vi "GetElevatorStatus.vi"(11 "Action":enum16{"Get", "Set", "Clear"}(ring)) -> (3 "Elevator Done?":bool)   [LabVIEW 2014, in "Elevator System.lvlib"]
uses:
  Elevator System.lvlib
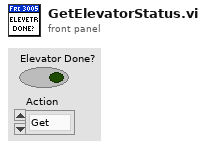
[diagram p1: front panel]
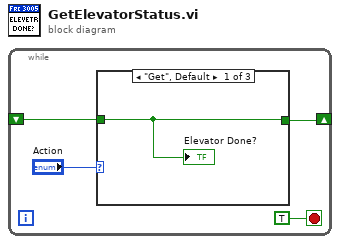
[diagram p0: block diagram]
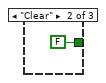
[diagram p2: hidden frame]
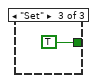
[diagram p3: hidden frame]
diagram:
  n1 = while {
    shift-right: [w2] -> _
    shift-left: _ -> [w1]
    stop <- TRUE stop-if-true
    n2 = case shown="\"Get\", Default" "Action" {
      tunnel: [w5 FALSE TRUE] -> w2
      tunnel: w1 -> [w5 _ _]
      frame "Get", Default {
        "Elevator Done?" <- w5
      }
      frame "Clear" {
      }
      frame "Set" {
      }
    }
  }
